vi "sub_Send-Serial.vi"(8 "error in":errorcluster) -> (0 "error out":errorcluster)   [LabVIEW 2019]
uses:
  Ctrl/cmd_ini-RW.ctl
  Ctrl/cmd_RW.ctl
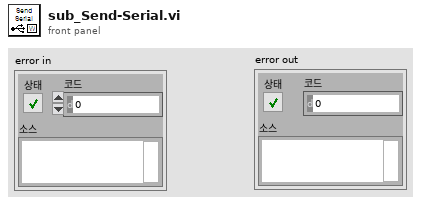
[diagram p1: front panel]
types:
  T1 = typedef "cmd_RW.ctl" = enum16{"read", "write"}
  T2 = typedef "cmd_ini-RW.ctl" = enum16{"ini", "read", "write"}
  T3 = cluster{"Ntrip tcp":bool, "GNSS serial":bool, "RTCM serial":bool, "Send serial":bool}
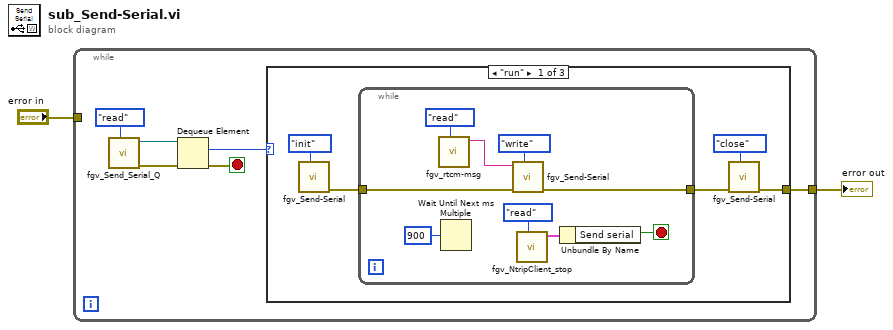
[diagram p0: block diagram]
diagram:
  n1 = while {
    tunnel: "error in" -> [_]
    tunnel: [w3] -> w1
    stop <- w4 stop-if-true
    n2 = call "fgv_Send_Serial_Q.vi"("cmd"=enum16{"create", "write", "read", "close"}."read") -> ("error out"=w6:errorcluster, "queue out"=w5:refnum<queue>)  [unwired: 9 in]
    n3 = Dequeue Element(queue=w5, error in (no error)=w6) -> (element=w8:enum16{"run", "check", "stop"}, error out=w4:errorcluster)  [unwired: 1 in, 2 out]
    n4 = case shown="\"run\"" w8 {
      tunnel: [w9 _ _] -> w3
      frame "run" {
        n5 = call "fgv_Send-Serial.vi"("cmd"=enum16{"init", "read", "write", "close"}."init") -> ("error out"=w12:errorcluster)  [unwired: 8 in, 2 out]
        n6 = while {
          tunnel: w12 -> [w17]
          tunnel: [w16] -> w10
          stop <- w19 stop-if-true
          n7 = call "fgv_rtcm-msg.vi"("cmd"=cmd_RW."read") -> ("rtcm msg out"=w14:string)  [unwired: 10 in]
          n8 = Wait Until Next ms Multiple(millisecond multiple=u32 900 ("ms 배수")) -> ()  [unwired: 1 out]
          n9 = call "fgv_Send-Serial.vi"("cmd"=enum16{"init", "read", "write", "close"}."write", "error in"=w17, "write buff"=w14) -> ("error out"=w16:errorcluster)  [unwired: 6 in, 2 out]
          n10 = call "fgv_NtripClient_stop.vi"("cmd"=cmd_ini-RW."read") -> ("local stops out"=w20:T3)  [unwired: 10 in]
          n11 = Unbundle By Name(w20) -> ("Send serial"=w19:bool)
        }
        n12 = call "fgv_Send-Serial.vi"("cmd"=enum16{"init", "read", "write", "close"}."close", "error in"=w10) -> ("error out"=w9:errorcluster)  [unwired: 7 in, 2 out]
      }
      frame "check" {
      }
      frame "stop", Default {
      }
    }
  }
  "error out" <- w1
